vi "Main.vi"(11 "Module Admin":refnum<class "Delacor_lib_QMH_Module Admin.lvclass">) -> ()   [LabVIEW 2020, in "ATM.lvlib"]
doc: "This template is based off of the Queued Message Handler design pattern and the Queued Message Handler project template that ships with LabVIEW.\n\nThe main difference is that the queue is private to this module and communication between modules is performed via Broadcast and Request events.\n\nRequest events are wrapped in public API methods and are handled in the Event Handling Loop (EHL) of this VI. Any module can register for Broadcast events sent by this module. The EHL generates messages based on user interface actions.\n\nThe Message Handling Loop (MHL) processes messages generated by the EHL, or by other messages. The messages are string values, so new messages can be added easily to the Message Cases case structure in the MHL. Each message cluster can also provide an optional value for Message Data, which is a variant that can be converted to whatever message-specific data is required.\n_____\nBased on DQMH Dev Tools: Project Template 7.1.0.1503."
uses:
  ATM.lvlib
  <vilib>/Delacor/Delacor QMH/Libraries/Message Queue_class/Delacor_lib_QMH_Message Queue.lvclass
  Module Data--cluster.ctl
  <vilib>/Utility/miscctls.llb/LVPointTypeDef.ctl
  <vilib>/Delacor/Delacor QMH/Libraries/Message Queue_class/Delacor_lib_QMH_Enqueue Message (Single).vi
  Stop Argument--cluster.ctl
  <vilib>/Delacor/Delacor QMH/Libraries/Module Admin_class/Delacor_lib_QMH_Module Admin.lvclass
  Update ATM Messages Argument--cluster.ctl
  Account Info -- cluster.ctl
  Deposit Introduced Argument--cluster.ctl
  Accounts Info -- cluster.ctl
  Check Withdrawal Argument--cluster.ctl
  <vilib>/ErrorRing/Error Ring.xnode
panel:
  in  "Enter":bool
  in  "User Input":string
  in  "Right Buttons":T1
  out "Right Menu":T2
  in  "Left Buttons":T1
  out "Left Menu":T2
  in  "Card Simulator":bool
  out "ATM Messages":string
  out "error out":errorcluster
  out "Status":string
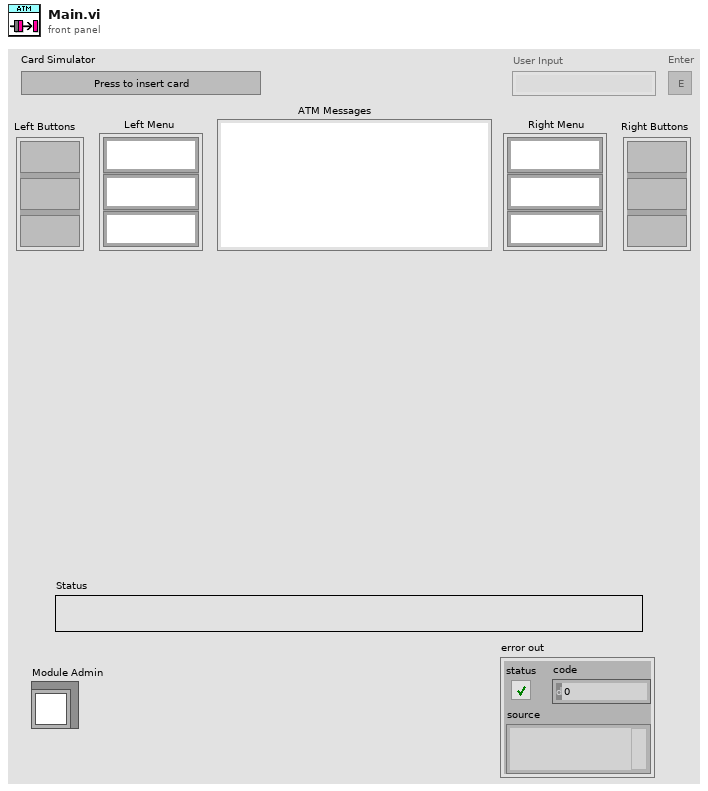
[diagram p1: front panel]
types:
  T1 = cluster{"Func Button":bool, "Func Button 2":bool, "Func Button 3":bool}
  T2 = cluster{"RFS String":string, "RFS String 2":string, "RFS String 3":string}
  T3 = typedef "ATM.lvlib/Request Events--cluster.ctl" = cluster{"Stop Module":refnum<user-event>, "Show Panel":refnum<user-event>, "Hide Panel":refnum<user-event>, "Get Module Execution Status":refnum<user-event>, "Show Diagram":refnum<user-event>, "Private.Set Up Controls":refnum<user-event>, "Private.Update ATM Messages":refnum<user-event>, "Private.Start Timeout":refnum<user-event>, "Private.Set Up Accounts File":refnum<user-event>, "Private.Verification OK":refnum<user-event>, "Private.Session Timed Out":refnum<user-event>, "Private.Verification NOK":refnum<user-event>, "Private.Stop Timeout":refnum<user-event>, "Private.Deposit Introduced":refnum<user-event>, "Private.Save Account":refnum<user-event>, "Private.Check Withdrawal":refnum<user-event>, "Testing - Update ATM Messages":refnum<user-event>, "Testing - Generate File Not Found Error":refnum<user-event>, "Testing - Enable All Elements in FP":refnum<user-event>, "Testing - Disable All Elements in FP":refnum<user-event>}
  T4 = typedef "ATM.lvlib/Module Data--cluster.ctl" = cluster{"Status":string, "User Input":string, "Verification OK?":bool, "User Input ref":refnum<vi>, "Left Buttons ref":refnum<vi>, "Right Buttons ref":refnum<vi>, "Enter ref":refnum<vi>, "Right Menu ref":refnum<vi>, "Left Menu ref":refnum<vi>, "Card Simulator":refnum<vi>, "Accounts.txt file name":string, "Accounts.txt file path":path, "Account Info":T5, "Accounts info":T6, "Pressed Button":string, "Index of Account":i32}
  T5 = typedef "ATM.lvlib/Account Info -- cluster.ctl" = cluster{"Account Number":string, "Name":string, "Surname":string, "Remaining Money":i32}
  T6 = typedef "ATM.lvlib/Accounts Info -- cluster.ctl" = T5[]
  T7 = typedef "ATM.lvlib/Check Withdrawal Argument--cluster.ctl" = cluster{"Withdraw Money":i32}
  T8 = typedef "ATM.lvlib/Deposit Introduced Argument--cluster.ctl" = cluster{"Deposit Money":u32}
  T9 = typedef "ATM.lvlib/Update ATM Messages Argument--cluster.ctl" = cluster{"ATM Messages":string}
  T10 = enum32{"invalid lock state", "Not Locked", "Locked (No Password)", "Password-protected"}
  T11 = typedef "ATM.lvlib/Stop Argument--cluster.ctl" = cluster{"Origin":string, "Exit via Stop Module Req?":bool, "Wait for Module to stop?":bool}
  T12 = typedef "LVPointTypeDef.ctl" = cluster{"Horizontal":i16, "Vertical":i16}
  T13 = enum32{"Invalid", "Standard", "Closed", "Hidden", "Minimized", "Maximized"}
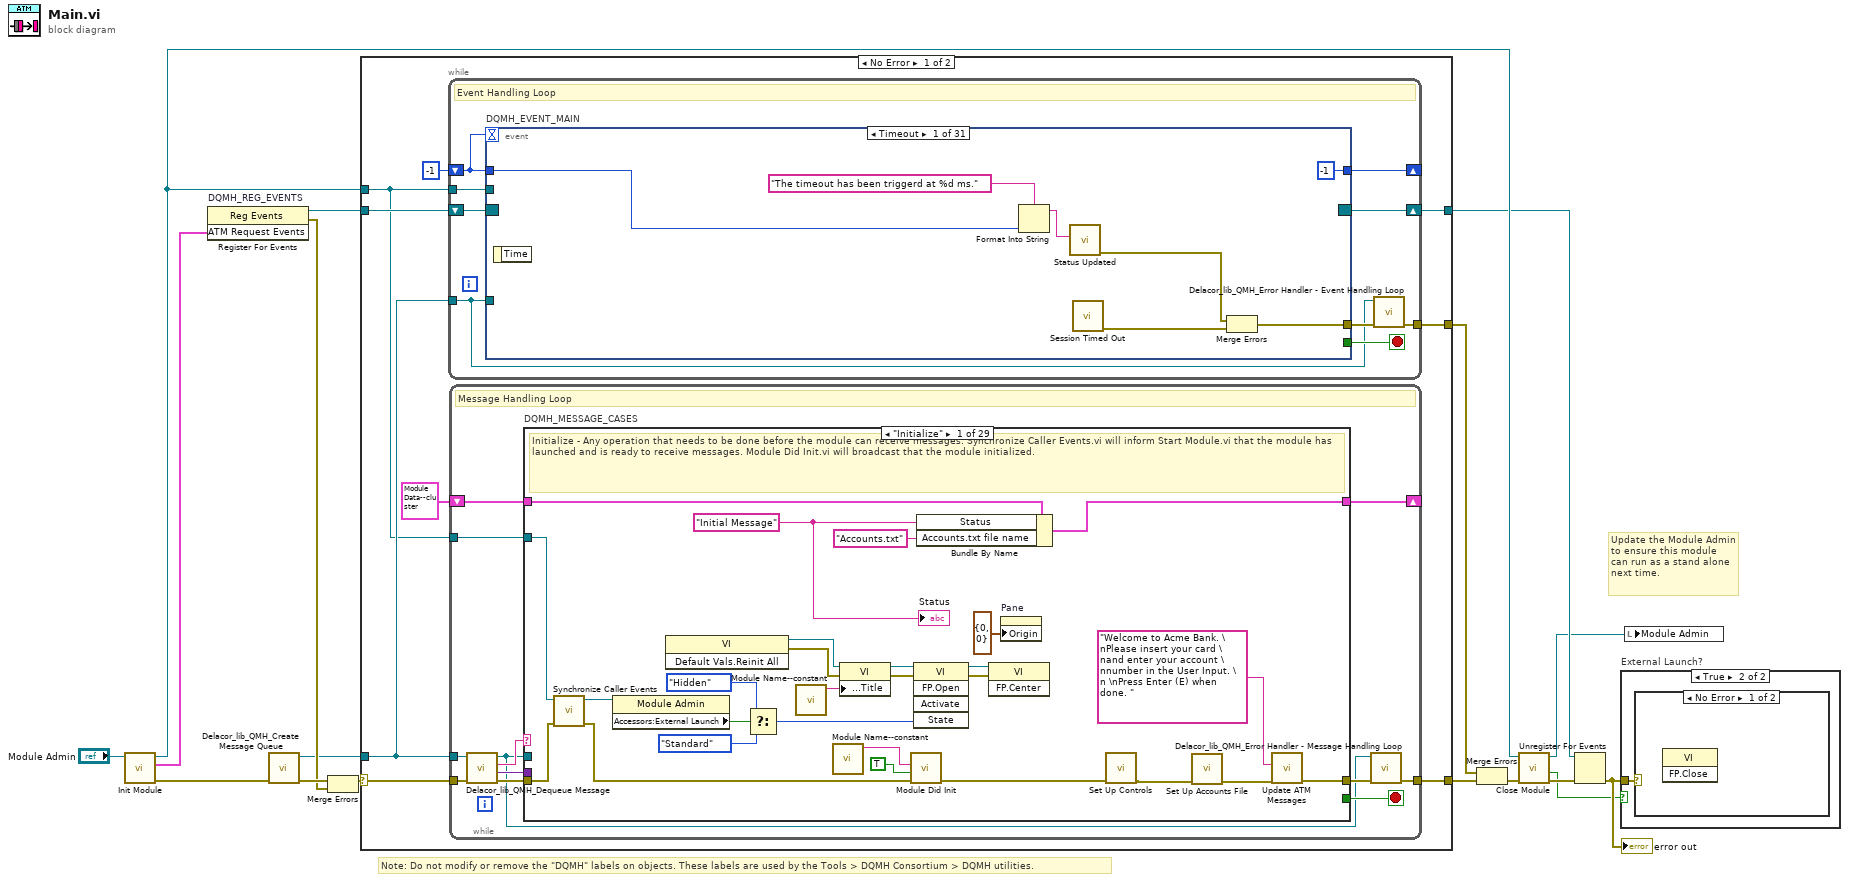
[diagram p0: block diagram]
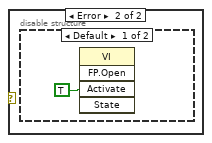
[diagram p3: hidden frame]
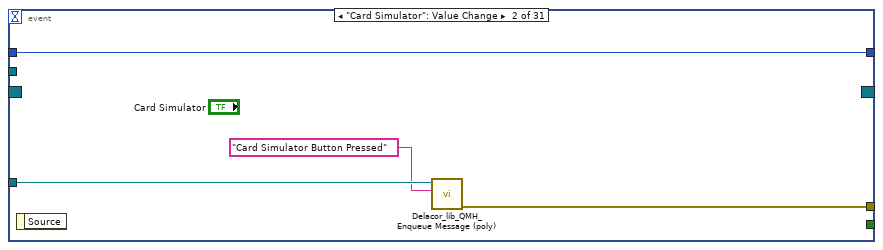
[diagram p5: hidden frame]
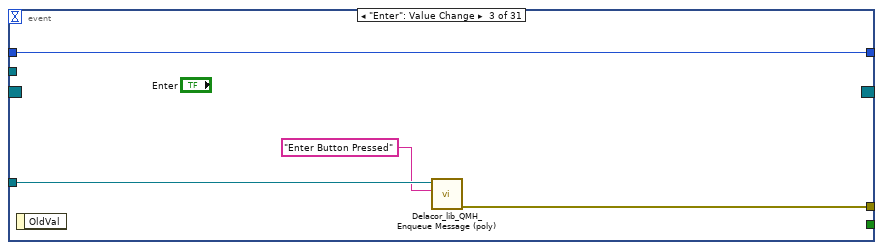
[diagram p6: hidden frame]
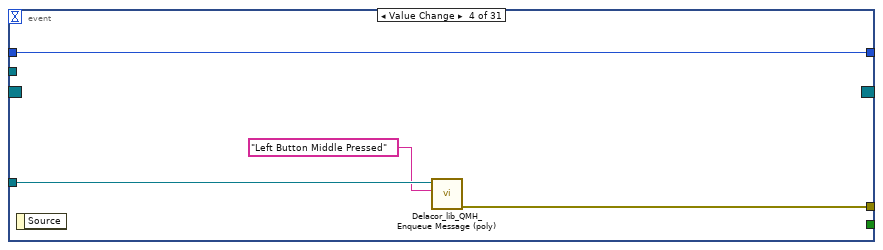
[diagram p7: hidden frame]
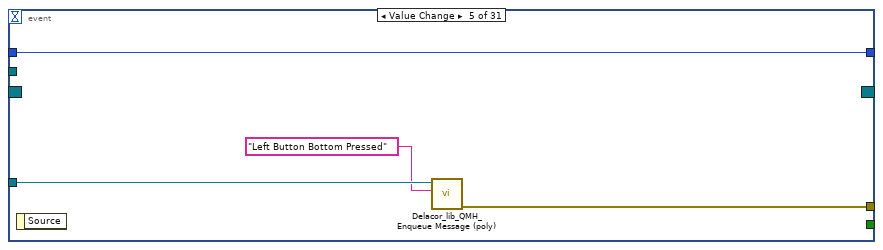
[diagram p8: hidden frame]
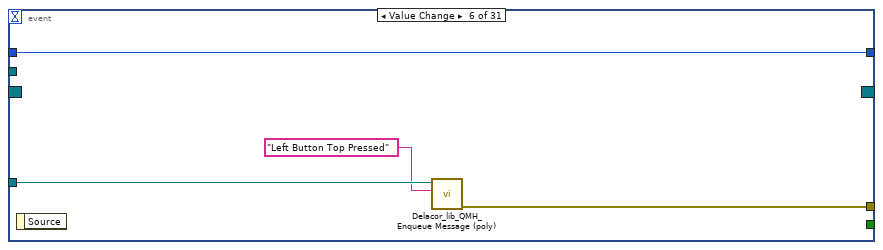
[diagram p9: hidden frame]
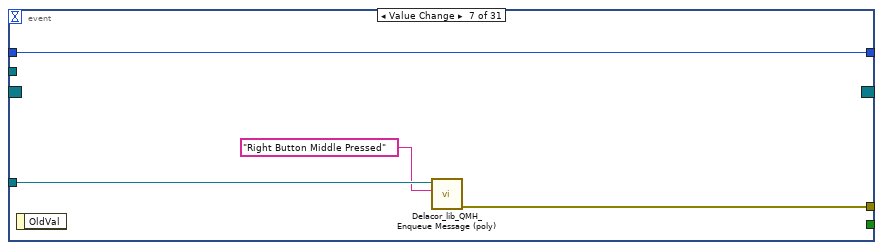
[diagram p10: hidden frame]
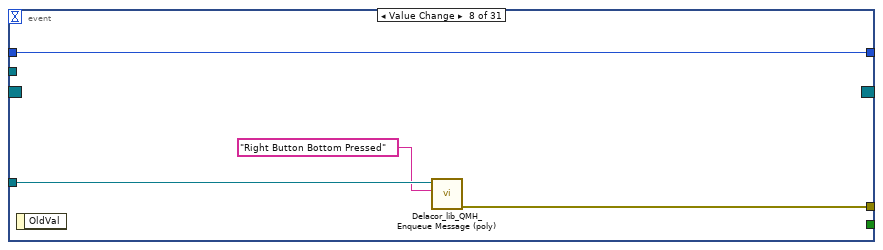
[diagram p11: hidden frame]
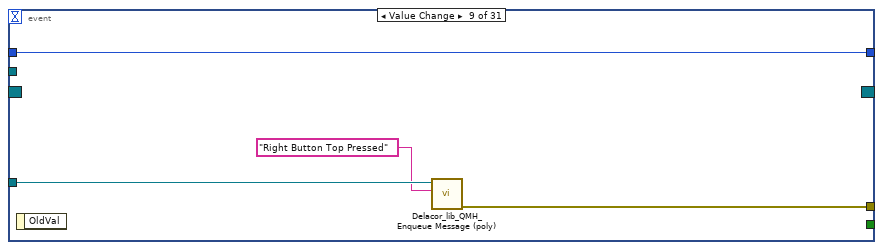
[diagram p12: hidden frame]
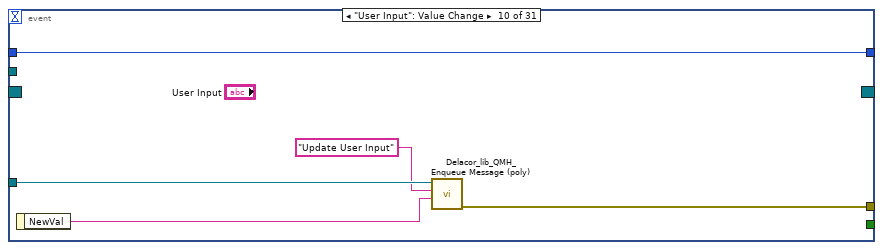
[diagram p13: hidden frame]
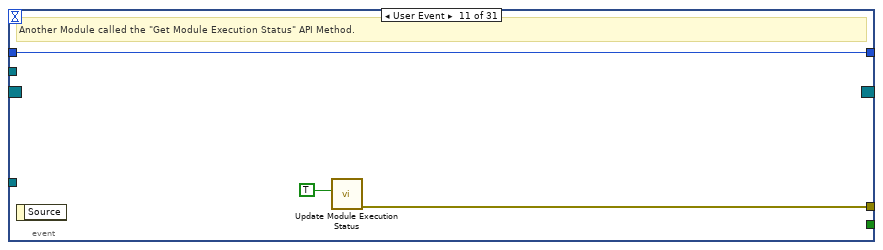
[diagram p14: hidden frame]
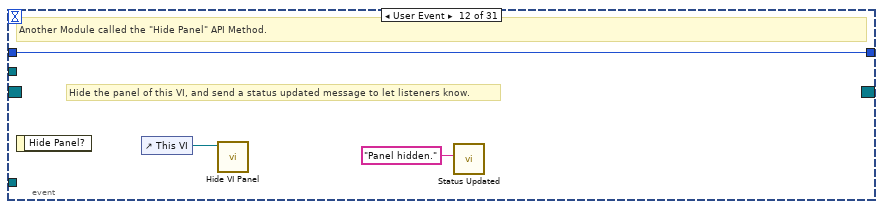
[diagram p15: hidden frame]
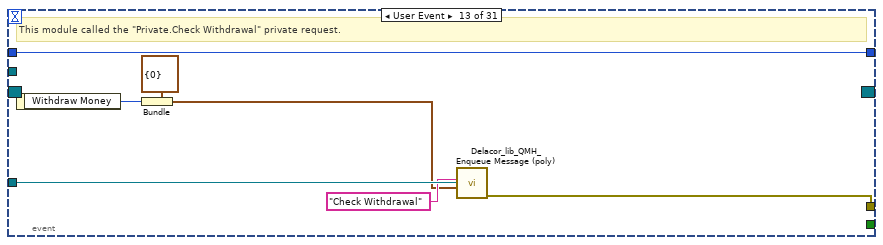
[diagram p16: hidden frame]
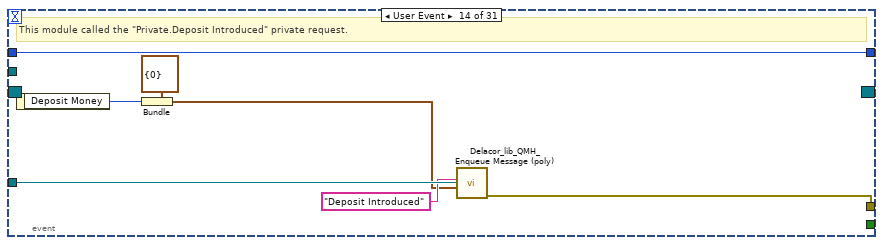
[diagram p17: hidden frame]
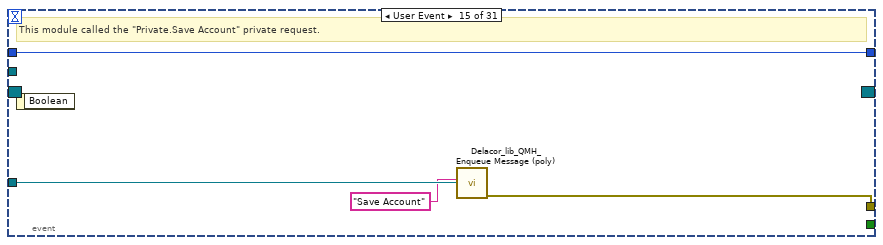
[diagram p18: hidden frame]
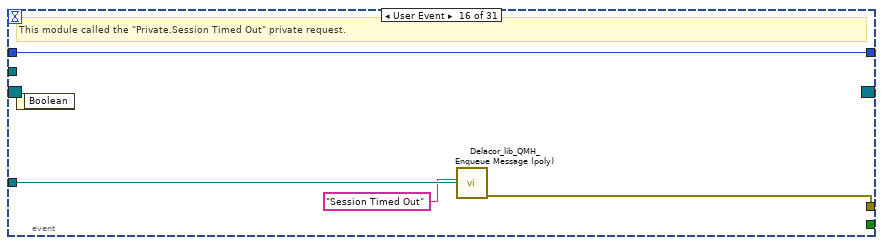
[diagram p19: hidden frame]
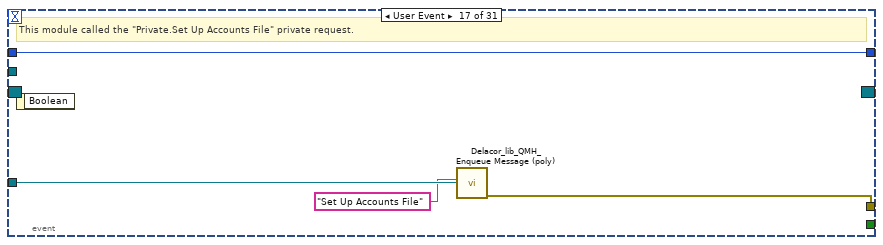
[diagram p20: hidden frame]
diagram:
  # "Note: Do not modify or remove the \"DQMH\" labels on objects. These labels are used by the Tools > DQMH Consortium > DQMH utilities."
  # "Update the Module Admin to ensure this module can run as a stand alone next time."
  n1 = call "Init Module.vi"("Singleton Module Admin in"="Module Admin") -> ("error out"=w16:errorcluster, "ATM Request Events"=w5:T3, "Singleton Module Admin out"=w8:refnum<class "Delacor_lib_QMH_Module Admin.lvclass">)  [unwired: 8 in]
  n2 = register-events "DQMH_REG_EVENTS"(w5) -> (reference out=w6:refnum<event-registration>, error out=w9:errorcluster)  [unwired: 2 in]
  n3 = call <vilib>:"Delacor_lib_QMH_Create Message Queue.vi"("error in"=w16) -> ("error out"=w11:errorcluster, "Message Queue"=w4:refnum<class "Delacor_lib_QMH_Message Queue.lvclass">)  [unwired: 9 in]
  n4 = Merge Errors(w11, w9) -> (w10:errorcluster)
  n5 = case shown="No Error" w10 {
    selector: w10 -> [w24 w589]
    tunnel: [w26 w588] -> w17
    tunnel: [w23 w587] -> w7
    tunnel: w6 -> [w21 w587]
    tunnel: w4 -> [w20 w582]
    tunnel: [w25 _] -> w14
    tunnel: w8 -> [w19 w583]
    frame No Error {
      n6 = while {
        tunnel: w20 -> [w29]
        shift-right: [w32] -> w23
        shift-left: w21 -> [w33]
        tunnel: [w34] -> w25
        tunnel: w19 -> [w30]
        shift-right: [w28] -> _
        shift-left: -1 ("Timeout Time") -> [w27]
        stop <- w31 stop-if-true
        # "Event Handling Loop"
        n7 = event "DQMH_EVENT_MAIN" shown="[0] Timeout" {
          selector: w33 -> [_ _ _ _ _ _ _ _ _ _ _ _ _ _ _ _ _ _ _ _ _ _ _ _ _ _ _ _ _ _ _]
          dyn-events: [_ _ _ _ _ _ _ _ _ _ _ _ _ _ _ _ _ _ _ _ _ _ _ _ _ _ _ _ _ _ _] -> w32
          timeout: w27 -> [_ _ _ _ _ _ _ _ _ _ _ _ _ _ _ _ _ _ _ _ _ _ _ _ _ _ _ _ _ _ _]
          tunnel: [_ _ _ _ _ _ _ _ _ _ _ _ _ _ _ _ _ _ _ _ _ _ _ _ _ TRUE ("Discard?") _ _ _ _ _] -> w31
          tunnel: w29 -> [_ w46 w50 w54 w58 w62 w66 w70 w74 w79 _ _ w91 w98 w102 w106 w111 w115 _ _ w128 w131 w136 _ _ w158 w165 w169 w173 w177 w182]
          tunnel: [w37 w44 w48 w52 w56 w60 w64 w68 w72 w77 w82 _ w86 w93 w100 w104 w109 w113 w120 _ w123 w129 w134 _ _ w161 w163 w167 w171 w175 w184] -> w35
          tunnel: w30 -> [_ _ _ _ _ _ _ _ _ _ _ _ _ _ _ _ _ _ _ _ _ _ _ _ _ _ _ _ _ _ w181]
          tunnel: [-1 ("Timeout Time") w43 w47 w51 w55 w59 w63 w67 w71 w75 w80 w83 w92 w99 w103 w107 w108 w112 w118 -1 ("Timeout Time") w122 w132 w133 w137 w147 w150 w166 w170 w174 w178 w179] -> w28
          tunnel: w27 -> [w39 w43 w47 w51 w55 w59 w63 w67 w71 w75 w80 w83 w92 w99 w103 w107 w108 w112 _ _ w122 w132 w133 w137 w147 w150 w166 w170 w174 w178 w179]
          event Timeout {
            n8 = event-data() -> ()  [unwired: 1 in, 1 out]
            n9 = Format Into String(format string="The timeout has been triggerd at %d ms.", w39) -> (resulting string=w38:string)  [unwired: 2 in, 1 out]
            n10 = call "Status Updated.vi"("Status"=w38) -> ("error out"=w36:errorcluster)  [unwired: 10 in]
            n11 = call "Session Timed Out.vi"() -> ("error out"=w41:errorcluster)  [unwired: 11 in]
            n12 = Merge Errors(w36, w41) -> (w37:errorcluster)
          }
          event "Card Simulator": Value Change {
            n13 = event-data() -> ()  [unwired: 1 in, 1 out]
            n14 = call-poly <vilib>:"Delacor_lib_QMH_Enqueue Message (poly).vi"("Message"="Card Simulator Button Pressed", "Message Queue in"=w46) -> ("error out"=w44:errorcluster)  [unwired: 8 in, 1 out]
          }
          event "Enter": Value Change {
            n15 = event-data() -> ()  [unwired: 1 in, 1 out]
            n16 = call-poly <vilib>:"Delacor_lib_QMH_Enqueue Message (poly).vi"("Message"="Enter Button Pressed", "Message Queue in"=w50) -> ("error out"=w48:errorcluster)  [unwired: 8 in, 1 out]
          }
          event "Left Buttons.Func Button 2": Value Change {
            n17 = event-data() -> ()  [unwired: 1 in, 1 out]
            n18 = call-poly <vilib>:"Delacor_lib_QMH_Enqueue Message (poly).vi"("Message"="Left Button Middle Pressed", "Message Queue in"=w54) -> ("error out"=w52:errorcluster)  [unwired: 8 in, 1 out]
          }
          event "Left Buttons.Func Button 3": Value Change {
            n19 = event-data() -> ()  [unwired: 1 in, 1 out]
            n20 = call-poly <vilib>:"Delacor_lib_QMH_Enqueue Message (poly).vi"("Message"="Left Button Bottom Pressed", "Message Queue in"=w58) -> ("error out"=w56:errorcluster)  [unwired: 8 in, 1 out]
          }
          event "Left Buttons.Func Button": Value Change {
            n21 = event-data() -> ()  [unwired: 1 in, 1 out]
            n22 = call-poly <vilib>:"Delacor_lib_QMH_Enqueue Message (poly).vi"("Message"="Left Button Top Pressed", "Message Queue in"=w62) -> ("error out"=w60:errorcluster)  [unwired: 8 in, 1 out]
          }
          event "Right Buttons.Func Button 2": Value Change {
            n23 = event-data() -> ()  [unwired: 1 in, 1 out]
            n24 = call-poly <vilib>:"Delacor_lib_QMH_Enqueue Message (poly).vi"("Message"="Right Button Middle Pressed", "Message Queue in"=w66) -> ("error out"=w64:errorcluster)  [unwired: 8 in, 1 out]
          }
          event "Right Buttons.Func Button 3": Value Change {
            n25 = event-data() -> ()  [unwired: 1 in, 1 out]
            n26 = call-poly <vilib>:"Delacor_lib_QMH_Enqueue Message (poly).vi"("Message"="Right Button Bottom Pressed", "Message Queue in"=w70) -> ("error out"=w68:errorcluster)  [unwired: 8 in, 1 out]
          }
          event "Right Buttons.Func Button": Value Change {
            n27 = event-data() -> ()  [unwired: 1 in, 1 out]
            n28 = call-poly <vilib>:"Delacor_lib_QMH_Enqueue Message (poly).vi"("Message"="Right Button Top Pressed", "Message Queue in"=w74) -> ("error out"=w72:errorcluster)  [unwired: 8 in, 1 out]
          }
          event "User Input": Value Change {
            n29 = event-data() -> ("NewVal"=w76:string)  [unwired: 1 in]
            n30 = call-poly <vilib>:"Delacor_lib_QMH_Enqueue Message (poly).vi"("Message Data"=w76, "Message"="Update User Input", "Message Queue in"=w79) -> ("error out"=w77:errorcluster)  [unwired: 7 in, 1 out]
          }
          event User Event {
            # "Another Module called the \"Get Module Execution Status\" API Method."
            n31 = event-data() -> ()  [unwired: 1 in, 1 out]
            n32 = call "Update Module Execution Status.vi"("Running?"=TRUE) -> ("error out"=w82:errorcluster)  [unwired: 10 in]
          }
          event User Event {
            # "Hide the panel of this VI, and send a status updated message to let listeners know."
            # "Another Module called the \"Hide Panel\" API Method."
            n33 = event-data() -> ()  [unwired: 1 in, 1 out]
            n34 = control-ref of="This VI"() -> (w85:refnum<vi>)
            n35 = call "Hide VI Panel.vi"("VI"=w85) -> ()  [unwired: 10 in, 1 out]
            n36 = call "Status Updated.vi"("Status"="Panel hidden." ("format string")) -> ()  [unwired: 10 in, 1 out]
          }
          event User Event {
            # "This module called the \"Private.Check Withdrawal\" private request."
            n37 = event-data() -> ("Withdraw Money"=w87:i32)  [unwired: 1 in]
            n38 = Bundle(cluster=T7 {"Withdraw Money"=0} ("Check Withdrawal Argument"), "Withdraw Money"=w87) -> (w88:T7)
            n39 = call-poly <vilib>:"Delacor_lib_QMH_Enqueue Message (poly).vi"("Message Data"=w88, "Message"="Check Withdrawal", "Message Queue in"=w91) -> ("error out"=w86:errorcluster)  [unwired: 7 in, 1 out]
          }
          event User Event {
            # "This module called the \"Private.Deposit Introduced\" private request."
            n40 = event-data() -> ("Deposit Money"=w94:u32)  [unwired: 1 in]
            n41 = Bundle(cluster=T8 {"Deposit Money"=0} ("Deposit Introduced Argument"), "Deposit Money"=w94) -> (w95:T8)
            n42 = call-poly <vilib>:"Delacor_lib_QMH_Enqueue Message (poly).vi"("Message Data"=w95, "Message"="Deposit Introduced", "Message Queue in"=w98) -> ("error out"=w93:errorcluster)  [unwired: 7 in, 1 out]
          }
          event User Event {
            # "This module called the \"Private.Save Account\" private request."
            n43 = event-data() -> ()  [unwired: 1 in, 1 out]
            n44 = call-poly <vilib>:"Delacor_lib_QMH_Enqueue Message (poly).vi"("Message"="Save Account", "Message Queue in"=w102) -> ("error out"=w100:errorcluster)  [unwired: 8 in, 1 out]
          }
          event User Event {
            # "This module called the \"Private.Session Timed Out\" private request."
            n45 = event-data() -> ()  [unwired: 1 in, 1 out]
            n46 = call-poly <vilib>:"Delacor_lib_QMH_Enqueue Message (poly).vi"("Message"="Session Timed Out", "Message Queue in"=w106) -> ("error out"=w104:errorcluster)  [unwired: 8 in, 1 out]
          }
          event User Event {
            # "This module called the \"Private.Set Up Accounts File\" private request."
            n47 = event-data() -> ()  [unwired: 1 in, 1 out]
            n48 = call-poly <vilib>:"Delacor_lib_QMH_Enqueue Message (poly).vi"("Message"="Set Up Accounts File", "Message Queue in"=w111) -> ("error out"=w109:errorcluster)  [unwired: 8 in, 1 out]
          }
          event User Event {
            # "This module called the \"Private.Set Up Controls\" private request."
            n49 = event-data() -> ()  [unwired: 1 in, 1 out]
            n50 = call-poly <vilib>:"Delacor_lib_QMH_Enqueue Message (poly).vi"("Message"="Set Up Controls", "Message Queue in"=w115) -> ("error out"=w113:errorcluster)  [unwired: 8 in, 1 out]
          }
          event User Event {
            # "This module called the \"Private.Start Timeout\" private request."
            n51 = event-data() -> ("Timeout Time"=w118:i32)  [unwired: 1 in]
            n52 = Format Into String(format string="A Timeout has been launched with a value of %d ms.", w118) -> (resulting string=w117:string, error out=w116:errorcluster)  [unwired: 2 in]
            n53 = call "Status Updated.vi"("error in"=w116, "Status"=w117) -> ("error out"=w120:errorcluster)  [unwired: 9 in]
          }
          event User Event {
            # "This module called the \"Private.Stop Timeout\" private request."
            n54 = event-data() -> ()  [unwired: 1 in, 1 out]
          }
          event User Event {
            # "This module called the \"Private.Update ATM Messages\" private request."
            n55 = event-data() -> ("ATM Messages"=w124:string)  [unwired: 1 in]
            n56 = Bundle(cluster=T9 {"ATM Messages"=""} ("Update ATM Messages Argument"), "ATM Messages"=w124) -> (w125:T9)
            n57 = call-poly <vilib>:"Delacor_lib_QMH_Enqueue Message (poly).vi"("Message Data"=w125, "Message"="Update ATM Messages", "Message Queue in"=w128) -> ("error out"=w123:errorcluster)  [unwired: 7 in, 1 out]
          }
          event User Event {
            # "This module called the \"Private.Verification NOK\" private request."
            n58 = event-data() -> ()  [unwired: 1 in, 1 out]
            n59 = call-poly <vilib>:"Delacor_lib_QMH_Enqueue Message (poly).vi"("Message"="Verification NOK", "Message Queue in"=w131) -> ("error out"=w129:errorcluster)  [unwired: 8 in, 1 out]
          }
          event User Event {
            # "This module called the \"Private.Verification OK\" private request."
            n60 = event-data() -> ()  [unwired: 1 in, 1 out]
            n61 = call-poly <vilib>:"Delacor_lib_QMH_Enqueue Message (poly).vi"("Message"="Verification OK", "Message Queue in"=w136) -> ("error out"=w134:errorcluster)  [unwired: 8 in, 1 out]
          }
          event User Event {
            # "Another Module called the \"Show Diagram\" API Method. This event is used for debugging."
            n62 = event-data() -> ()  [unwired: 1 in, 1 out]
            n63 = disable-structure shown="RUN_TIME_ENGINE==False" {
              frame condition #0 (active) {
                # "functionality not available in exe"
                n64 = invoke on="Invoke Node" class="VI" method="Lock State.Get"() -> (error out=w143:errorcluster, "Get Lock State"=w142:T10, "pwd in cache"=w139:bool)  [unwired: 4 in, 1 out]
                n65 = Equal?(x=T10."Password-protected", y=w142) -> (x = y?=w140:bool)
                n66 = Compound Arithmetic op=AND(w140, invert w139) -> (w138:bool)
                n67 = case shown="False" w138 {
                  tunnel: w143 -> [w146 _]
                  frame False {
                    n68 = property on="Property Node" class="VI"(error in=w146, "BDWin.Open"=TRUE ("Block Diagram Window:Open")) -> ()  [unwired: 1 in, 2 out]
                    n69 = call "Status Updated.vi"("Status"="Block Diagram shown." ("format string")) -> ()  [unwired: 10 in, 1 out]
                  }
                  frame True {
                    # "Password-protected VI, and the password is not in the cache. Do not show the diagram."
                  }
                }
              }
              frame condition #1 {
              }
            }
          }
          event User Event {
            # "Show the panel of this VI, and send a status updated message to let listeners know."
            # "Another Module called the \"Show Panel\" API Method."
            n70 = event-data() -> ()  [unwired: 1 in, 1 out]
            n71 = control-ref of="This VI"() -> (w149:refnum<vi>)
            n72 = call "Open VI Panel.vi"("VI"=w149) -> ()  [unwired: 10 in, 1 out]
            n73 = call "Status Updated.vi"("Status"="Panel shown." ("format string")) -> ()  [unwired: 10 in, 1 out]
          }
          event User Event {
            # "The Stop Module Event can get fired from the Exit message in the MHL. The queue gets destroyed in that case. If the queue no longer exists, the Enqueue Exit as a priority message will return error 1. It is safe to ignore, because the module is already exiting."
            # "Another Module called the \"Stop Module\" API Method  or the Message Handling Loop below."
            n74 = event-data() -> ("Origin"=w157:string, "Exit via Stop Module Req?"=w153:bool, "Wait for Module to stop?"=w152:bool)  [unwired: 1 in]
            n75 = local write "Status"(w157) -> ()
            n76 = Bundle By Name(cluster=T11 {"Origin"="", "Exit via Stop Module Req?"=FALSE, "Wait for Module to stop?"=FALSE} ("Stop Argument"), "Exit via Stop Module Req?"=w153, "Wait for Module to stop?"=w152) -> (w151:T11)
            n77 = call-poly <vilib>:"Delacor_lib_QMH_Enqueue Message (poly).vi"("Priority Message? (F)"=TRUE, "Message Data"=w151, "Message"="Exit", "Message Queue in"=w158) -> ("error out"=w162:errorcluster)  [unwired: 6 in, 1 out]
            n78 = call <vilib>:"Clear Errors.vi"("error in (no error)"=w162, "specific error code to clear (0: all)"=1) -> ("error out"=w161:errorcluster)  [unwired: 4 in, 1 out]
          }
          event User Event {
            # "Another Module called the \"Testing - Disable All Elements in FP\" API Method."
            n79 = event-data() -> ()  [unwired: 1 in, 1 out]
            n80 = call-poly <vilib>:"Delacor_lib_QMH_Enqueue Message (poly).vi"("Message"="Testing - Disable All Elements in FP", "Message Queue in"=w165) -> ("error out"=w163:errorcluster)  [unwired: 8 in, 1 out]
          }
          event User Event {
            # "Another Module called the \"Testing - Enable All Elements in FP\" API Method."
            n81 = event-data() -> ()  [unwired: 1 in, 1 out]
            n82 = call-poly <vilib>:"Delacor_lib_QMH_Enqueue Message (poly).vi"("Message"="Testing - Enable All Elements in FP", "Message Queue in"=w169) -> ("error out"=w167:errorcluster)  [unwired: 8 in, 1 out]
          }
          event User Event {
            # "Another Module called the \"Testing - Generate File Not Found Error\" API Method."
            n83 = event-data() -> ()  [unwired: 1 in, 1 out]
            n84 = call-poly <vilib>:"Delacor_lib_QMH_Enqueue Message (poly).vi"("Message"="Testing - Generate File Not Found Error", "Message Queue in"=w173) -> ("error out"=w171:errorcluster)  [unwired: 8 in, 1 out]
          }
          event User Event {
            # "Another Module called the \"Testing - Update ATM Messages\" API Method."
            n85 = event-data() -> ()  [unwired: 1 in, 1 out]
            n86 = call-poly <vilib>:"Delacor_lib_QMH_Enqueue Message (poly).vi"("Message"="Testing - Update ATM Messages", "Message Queue in"=w177) -> ("error out"=w175:errorcluster)  [unwired: 8 in, 1 out]
          }
          event Panel Close? {
            w183 = TRUE  # Discard the event, the MHL is responsible for closing and stopping this VI.
            # "Hide the panel or send the 'Exit' message if the user clicks the 'X' on the module main VI panel."
            n87 = event-data() -> ()  [unwired: 1 in, 1 out]
            n88 = property on="Property Node" class="Module Admin"(reference=w181) -> ("Accessors:External Launch"=w180:bool)  [unwired: 1 in, 2 out]
            n89 = case shown="True" w180 {
              tunnel: w182 -> [_ w190]
              tunnel: [_ w191] -> w184
              frame True {
                # "If externally launched, clicking the 'X' hides the panel, but doesn't close it."
                n90 = control-ref of="This VI"() -> (w187:refnum<vi>)
                n91 = call "Hide VI Panel.vi"("VI"=w187) -> ("error out"=w185:errorcluster)  [unwired: 10 in]
                n92 = call "Status Updated.vi"("error in"=w185, "Status"="Panel hidden." ("format string")) -> ()  [unwired: 9 in, 1 out]
              }
              frame False {
                # "If run as a stand-alone VI, clicking the panel 'X' stops the VI."
                n93 = call-poly <vilib>:"Delacor_lib_QMH_Enqueue Message (poly).vi"("Priority Message? (F)"=TRUE, "Message"="Exit", "Message Queue in"=w190) -> ("error out"=w191:errorcluster)  [unwired: 7 in, 1 out]
              }
            }
            n94 = event-data ("Event Filter Node")("Discard?"=w183) -> ()  [unwired: 1 in, 1 out]
          }
        }
        n95 = call-dynamic "Delacor_lib_QMH_Error Handler - Event Handling Loop.vi"("error in"=w35, "Message Queue in"=w29) -> ("dup error in"=w34:errorcluster)  [unwired: 8 in, 1 out]
      }
      n96 = while {
        tunnel: w20 -> [w192]
        shift-right: [w200] -> _
        shift-left: T4 {"Status"="", "User Input"="", "Verification OK?"=FALSE, "User Input ref"=refnum, "Left Buttons ref"=refnum, "Right Buttons ref"=refnum, "Enter ref"=refnum, "Right Menu ref"=refnum, "Left Menu ref"=refnum, "Card Simulator"=refnum, "Accounts.txt file name"="", "Accounts.txt file path"=path "", "Account Info"={"Account Number"="", "Name"="", "Surname"="", "Remaining Money"=0}, "Accounts info"=[], "Pressed Button"="", "Index of Account"=0} ("Data Cluster") -> [w201]
        tunnel: w24 -> [w203]
        tunnel: [w195] -> w26
        tunnel: w19 -> [w196]
        stop <- w199 stop-if-true
        # "Message Handling Loop"
        n97 = call-dynamic "Delacor_lib_QMH_Dequeue Message.vi"("error in"=w203, "Message Queue in"=w192) -> ("error out"=w202:errorcluster, "Message Data"=w197:variant, "Message"=w198:string, "Message Queue out"=w193:refnum<class "Delacor_lib_QMH_Message Queue.lvclass">)  [unwired: 6 in]
        n98 = case "DQMH_MESSAGE_CASES" shown="\"Initialize\"" w198 {
          selector: w198 -> [_ _ _ _ _ _ _ _ _ _ _ _ w367 w389 w399 w412 w421 _ _ _ _ _ _ _ _ _ _ _ w577]
          tunnel: w193 -> [_ _ _ _ _ _ _ _ _ _ _ _ _ _ _ _ _ _ _ _ _ _ _ _ _ _ w542 w565 _]
          tunnel: w202 -> [w228 w232 w247 w253 w264 w277 w292 w298 w301 w308 w322 w365 w378 w387 w398 w410 w418 w444 w453 w468 w490 w495 w499 w515 w531 w538 w549 w571 w580]
          tunnel: [w210 w232 w238 w252 w262 w279 w295 w297 w301 w306 w312 w358 w370 w391 w401 w414 w419 w428 w448 w462 w489 w492 w498 w514 w530 w538 w545 w566 w581] -> w194
          tunnel: w201 -> [w218 w231 w249 w257 w263 w289 w294 w299 w300 w307 w321 w364 w376 w384 w396 w407 w420 w440 w452 w459 w488 w496 w500 w513 w529 w537 w544 w564 w578]
          tunnel: [w217 w231 w248 w256 w263 w273 w294 w299 w300 w304 w318 w364 w368 w390 w400 w413 w422 w438 w447 w457 w488 w496 w500 w513 w529 w537 w544 w564 w578] -> w200
          tunnel: [_ _ _ _ _ _ _ _ _ _ _ _ _ _ _ _ _ _ _ _ _ _ _ _ _ _ _ w563 _] -> w199
          tunnel: w197 -> [_ _ _ _ w261 _ _ _ _ w305 _ _ _ _ _ _ _ w443 _ w467 _ _ _ _ _ _ w543 w562 _]
          tunnel: w196 -> [w219 _ _ _ _ _ _ _ _ _ _ _ _ _ _ _ _ _ _ _ _ _ _ _ _ _ w541 w557 _]
          frame "Initialize" {
            w213 = "Initial Message" ("Initial Message")
            # "Initialize - Any operation that needs to be done before the module can receive messages. Synchronize Caller Events.vi will inform Start Module.vi that the module has launched and is ready to receive messages. Module Did Init.vi will broadcast that the module initialized."
            n99 = call "Synchronize Caller Events.vi"("error in"=w228, "Singleton Module Admin in"=w219) -> ("error out"=w227:errorcluster, "Singleton Module Admin out"=w214:refnum<class "Delacor_lib_QMH_Module Admin.lvclass">)  [unwired: 8 in]
            n100 = property on="Property Node" class="Module Admin"(reference=w214) -> ("Accessors:External Launch"=w223:bool)  [unwired: 1 in, 2 out]
            n101 = invoke class="VI" method="Default Vals.Reinit All"() -> (reference out=w208:refnum<vi>, error out=w207:errorcluster)  [unwired: 3 in, 1 out]
            n102 = Select(t=T13."Hidden" ("State"), s=w223, f=T13."Standard" ("State")) -> (s? t:f=w220:T13)
            n103 = call "Module Name--constant.vi"() -> ("Module Name"=w226:string)  [unwired: 11 in]
            n104 = call "Module Name--constant.vi"() -> ("Module Name"=w215:string)  [unwired: 11 in]
            n105 = property on="Property Node" class="VI"(reference=w208, error in=w207, "Front Panel.Title"=w226) -> (reference out=w225:refnum<vi>, error out=w230:errorcluster)
            n106 = call "Module Did Init.vi"("error in"=w227, "Initialized?"=TRUE, "Origin"=w215) -> ("error out"=w211:errorcluster)  [unwired: 8 in]
            n107 = invoke on="Invoke Node" class="VI" method="FP.Open"(reference=w225, error in=w230, "State"=w220) -> (reference out=w224:refnum<vi>, error out=w229:errorcluster)  [unwired: 2 in, 3 out]
            n108 = Bundle By Name(cluster=w218, "Status"=w213, "Accounts.txt file name"="Accounts.txt") -> (w217:T4)
            n109 = invoke on="Invoke Node" class="VI" method="FP.Center"(reference=w224, error in=w229) -> ()  [unwired: 1 in, 3 out]
            n110 = property on="Pane" class="Pane"("Origin"=T12 {"Horizontal"=0, "Vertical"=0}) -> ()  [unwired: 2 in, 2 out]
            n111 = call "Set Up Controls.vi"("error in"=w211) -> ("error out"=w205:errorcluster)  [unwired: 10 in]
            n112 = call "Set Up Accounts File.vi"("error in"=w205) -> ("error out"=w204:errorcluster)  [unwired: 10 in]
            n113 = call "Update ATM Messages.vi"("error in"=w204, "ATM Messages"="Welcome to Acme Bank. \nPlease insert your card \nand enter your account \nnumber in the User Input. \n \nPress Enter (E) when done. " ("Initial Message")) -> ("error out"=w210:errorcluster)  [unwired: 9 in]
            "Status" <- w213
          }
          frame "--- Private Requests ---" {
          }
          frame "Set Up Controls" {
            w235 = FALSE  # Disabled&GrayOut
            n114 = control-ref of="Card Simulator"() -> (w239:refnum<vi>)
            n115 = control-ref of="User Input"() -> (w246:refnum<vi>)
            n116 = control-ref of="Right Buttons"() -> (w245:refnum<vi>)
            n117 = control-ref of="Left Buttons"() -> (w244:refnum<vi>)
            n118 = control-ref of="Enter"() -> (w243:refnum<vi>)
            n119 = control-ref of="Left Menu"() -> (w242:refnum<vi>)
            n120 = control-ref of="Right Menu"() -> (w241:refnum<vi>)
            n121 = Build Array(w246, w245, w244, w243, w242, w241) -> (w240:refnum<vi>[])
            n122 = Bundle By Name(cluster=w249, "User Input ref"=w246, "Left Buttons ref"=w245, "Right Buttons ref"=w244, "Enter ref"=w243, "Right Menu ref"=w242, "Left Menu ref"=w241, "Card Simulator"=w239) -> (w248:T4)
            n123 = call "Enable or disable control or indicators.vi"("Enable (T)/Disable&GrayOut (F)"=w235, "error in (no error)"=w247, "aray of references in"=w240) -> ("error out"=w237:errorcluster, "Array of references dup"=w236:refnum<vi>[])  [unwired: 7 in]
            n124 = call "Get Controls Indicators Status by name.vi"("Enable (T)/Disable&GrayOut (F)"=w235, "error in (no error)"=w237, "aray of references"=w236) -> ("error out"=w233:errorcluster, "Status description"=w234:string)  [unwired: 7 in]
            n125 = call "Status Updated.vi"("error in"=w233, "Status"=w234) -> ("error out"=w238:errorcluster)  [unwired: 9 in]
          }
          frame "Set Up Accounts File" {
            n126 = Unbundle By Name(w257) -> ("Accounts.txt file name"=w254:string)
            n127 = call <vilib>:"Application Directory.vi"() -> ("Application Directory"=w255:path)
            n128 = Build Path(base path=w255, name or relative path=w254) -> (appended path=w251:path)
            n129 = call "Read Accounts Data.vi"("error in (no error)"=w253, "Accounts.txt file path"=w251) -> ("error out"=w252:errorcluster, "Accounts info"=w250:T6)  [unwired: 8 in]
            n130 = Bundle By Name(cluster=w257, "Accounts.txt file path"=w251, "Accounts info"=w250) -> (w256:T4)
          }
          frame "Update ATM Messages" {
            n131 = Variant To Data(error in=w264, type=T9 {"ATM Messages"=""} ("Update ATM Messages Argument"), Variant=w261) -> (data=w259:T9, error out=w262:errorcluster)
            n132 = Unbundle By Name(w259) -> ("ATM Messages"=→"ATM Messages":string)
          }
          frame "Verification OK" {
            w270 = FALSE  # Disable&GrayOut
            w283 = TRUE  # Enable
            # "The introduced value as a account number is correct"
            n133 = Unbundle By Name(w289) -> ("Account Info.Name"=w287:string, "Account Info.Surname"=w286:string, "Left Buttons ref"=w282:refnum<vi>, "Right Buttons ref"=w281:refnum<vi>, "Left Menu ref"=w274:refnum<vi>, "Right Menu ref"=w275:refnum<vi>, "Enter ref"=w269:refnum<vi>, "User Input ref"=w265:refnum<vi>)
            n134 = Build Array(w282, w281, w274, w275) -> (w284:refnum<vi>[])
            n135 = call "Prepare Left and Right Menus Strings.vi"("error in (no error)"=w277, "Right Menu ref"=w274, "Left Menu ref"=w275) -> ("error out"=w276:errorcluster)  [unwired: 8 in]
            n136 = Build Array(w269, w265) -> (w268:refnum<vi>[])
            n137 = call "Enable or disable control or indicators.vi"("Enable (T)/Disable&GrayOut (F)"=w283, "error in (no error)"=w276, "aray of references in"=w284) -> ("error out"=w267:errorcluster)  [unwired: 7 in, 1 out]
            n138 = invoke class="Str" method="Reinit To Default"(reference=w265, error in=w267) -> (error out=w266:errorcluster)  [unwired: 1 in, 2 out]
            n139 = Format Into String(format string="Welcome to Acme Bank \n%s %s\n \nPlease select transaction \nby using the buttons. ", w287, w286) -> (resulting string=w285:string)  [unwired: 2 in, 1 out]
            n140 = call "Enable or disable control or indicators.vi"("Enable (T)/Disable&GrayOut (F)"=w270, "error in (no error)"=w266, "aray of references in"=w268) -> ("error out"=w271:errorcluster)  [unwired: 7 in, 1 out]
            n141 = Bundle By Name(cluster=w289, "Verification OK?"=TRUE) -> (w273:T4)
            n142 = call "Update ATM Messages.vi"("error in"=w271, "ATM Messages"=w285) -> ("error out"=w280:errorcluster)  [unwired: 9 in]
            n143 = call "Start Timeout.vi"("error in"=w280, "Timeout Time (ms)"=10000) -> ("error out"=w279:errorcluster)  [unwired: 9 in]
          }
          frame "Verification NOK" {
            w293 = TRUE  # Key Focus
            # "Focuses the cursor to the User Input control"
            # "The introduced value as a account number is incorrect"
            n144 = Unbundle By Name(w294) -> ("User Input ref"=w290:refnum<vi>)
            n145 = property class="Str"(reference=w290, error in=w292, "Key Focus"=w293) -> (error out=w291:errorcluster)  [unwired: 1 out]
            n146 = call "Update ATM Messages.vi"("error in"=w291, "ATM Messages"="Account Information Incorrect \nPlease Re-Enter Account Number. \nPress Enter (E) when done ") -> ("error out"=w295:errorcluster)  [unwired: 9 in]
          }
          frame "Session Timed Out" {
            # "If the session is inactive for 10 seconds, stops the application (The message has already been sent)."
            n147 = call "Stop Module.vi"("error in"=w298) -> ("error out"=w297:errorcluster)  [unwired: 10 in]
          }
          frame "--- User Interface Events ---" {
            # "The following states are for user interface events"
          }
          frame "Update User Input" {
            # "Receive the User Input and stores it in the Main Cluster"
            n148 = Variant To Data(error in=w308, type="", Variant=w305) -> (data=w303:string, error out=w306:errorcluster)
            n149 = Bundle By Name(cluster=w307, "User Input"=w303) -> (w304:T4)
          }
          frame "Enter Button Pressed" {
            w314 = 10000  # Timeout Time (ms)
            # "Receive the User Input and stores it in the Main Cluster"
            n150 = Unbundle By Name(w321) -> ("Index of Account"=w310:i32, "Account Info"=w316:T5, "Accounts info"=w320:T6, "User Input"=w319:string, "Verification OK?"=w315:bool, "Pressed Button"=w311:string)
            n151 = case shown="True" w315 {
              tunnel: w322 -> [w328 w341]
              tunnel: w320 -> [w327 _]
              tunnel: w319 -> [w326 w338]
              tunnel: [w325 w340] -> w313
              tunnel: [w324 w342] -> w317
              tunnel: w316 -> [_ w342]
              tunnel: w311 -> [_ w339]
              tunnel: w310 -> [_ w335]
              tunnel: [w323 w335] -> w309
              frame False {
                n152 = call "Get Account Info.vi"("error in (no error)"=w328, "Account Number"=w326, "Accounts info"=w327) -> ("error out"=w329:errorcluster, "Valid Account?"=w330:bool, "Account Info"=w324:T5, "Index of Account"=w323:i32)  [unwired: 5 in]
                n153 = case shown="False" w330 {
                  tunnel: w329 -> [w332 w334]
                  tunnel: [w331 w333] -> w325
                  frame False {
                    # "The Account does not exist"
                    n154 = call "Verification NOK.vi"("error in"=w332) -> ("error out"=w331:errorcluster)  [unwired: 10 in]
                  }
                  frame True {
                    # "The Account Exists"
                    n155 = call "Verification OK.vi"("error in"=w334) -> ("error out"=w333:errorcluster)  [unwired: 10 in]
                  }
                }
              }
              frame True {
                w336 = u32 0  # u32
                # "Already checked, deposit introduced"
                n156 = Decimal String To Number(string=w338, default (0L)=w336) -> (number=w337:u32)  [unwired: 1 in, 1 out]
                n157 = case shown="\"Right Button Middle Pressed\"" w339 {
                  tunnel: w341 -> [w345 w346 w347 w350]
                  tunnel: [w343 w346 w347 w349] -> w340
                  tunnel: w337 -> [w344 _ _ w348]
                  frame "Right Button Middle Pressed" {
                    # "Withdraw"
                    n158 = call "Check Withdrawal.vi"("error in"=w345, "Withdraw Money"=w344) -> ("error out"=w343:errorcluster)  [unwired: 9 in]
                  }
                  frame "Right Button Bottom Pressed" {
                    # "Fast Cash $50"
                  }
                  frame Default {
                  }
                  frame "Right Button Top Pressed" {
                    # "Deposit"
                    n159 = call "Deposit Introduced.vi"("error in"=w350, "Deposit Money"=w348) -> ("error out"=w349:errorcluster)  [unwired: 9 in]
                  }
                }
              }
            }
            n160 = Bundle By Name(cluster=w321, "Account Info"=w317, "Index of Account"=w309) -> (w318:T4)
            n161 = call "Start Timeout.vi"("error in"=w313, "Timeout Time (ms)"=w314) -> ("error out"=w312:errorcluster)  [unwired: 9 in]
          }
          frame "Card Simulator Button Pressed" {
            w361 = TRUE  # Key Focus
            w352 = TRUE  # Enabled
            # "Focuses the cursor to the User Input control"
            n162 = Unbundle By Name(w364) -> ("User Input ref"=w360:refnum<vi>, "Enter ref"=w363:refnum<vi>)
            n163 = Build Array(w360, w363) -> (w366:refnum<vi>[])
            n164 = Merge Errors(w365) -> (w362:errorcluster)
            n165 = call "Enable or disable control or indicators.vi"("Enable (T)/Disable&GrayOut (F)"=w352, "error in (no error)"=w362, "aray of references in"=w366) -> ("error out"=w356:errorcluster, "Array of references dup"=w353:refnum<vi>[])  [unwired: 7 in]
            n166 = call "Get Controls Indicators Status by name.vi"("Enable (T)/Disable&GrayOut (F)"=w352, "error in (no error)"=w356, "aray of references"=w353) -> ("error out"=w355:errorcluster, "Status description"=w357:string)  [unwired: 7 in]
            n167 = call "Status Updated.vi"("error in"=w355, "Status"=w357) -> ("error out"=w354:errorcluster)  [unwired: 9 in]
            n168 = property class="Str"(reference=w360, error in=w354, "Key Focus"=w361) -> (error out=w351:errorcluster)  [unwired: 1 out]
            n169 = call "Start Timeout.vi"("error in"=w351, "Timeout Time (ms)"=10000) -> ("error out"=w358:errorcluster)  [unwired: 9 in]
          }
          frame "Right Button Top Pressed" {
            w369 = 10000  # Timeout Time (ms)
            w377 = TRUE  # Enabled
            # "Deposit button pressed"
            n170 = Unbundle By Name(w376) -> ("Enter ref"=w375:refnum<vi>, "User Input ref"=w374:refnum<vi>)
            n171 = call "Update ATM Messages.vi"("error in"=w378, "ATM Messages"="Please enter amount to deposit and press \nEnter (E) when done ") -> ("error out"=w372:errorcluster)  [unwired: 9 in]
            n172 = Bundle By Name(cluster=w376, "Pressed Button"=w367) -> (w368:T4)
            n173 = Build Array(w375, w374) -> (w373:refnum<vi>[])
            n174 = call "Enable or disable control or indicators.vi"("Enable (T)/Disable&GrayOut (F)"=w377, "error in (no error)"=w372, "aray of references in"=w373) -> ("error out"=w371:errorcluster)  [unwired: 7 in, 1 out]
            n175 = call "Start Timeout.vi"("error in"=w371, "Timeout Time (ms)"=w369) -> ("error out"=w370:errorcluster)  [unwired: 9 in]
          }
          frame "Right Button Middle Pressed" {
            w388 = TRUE  # Enabled
            w392 = 10000  # Timeout Time (ms)
            # "Withdraw button pressed"
            n176 = Unbundle By Name(w384) -> ("Enter ref"=w386:refnum<vi>, "User Input ref"=w385:refnum<vi>)
            n177 = Build Array(w386, w385) -> (w383:refnum<vi>[])
            n178 = call "Enable or disable control or indicators.vi"("Enable (T)/Disable&GrayOut (F)"=w388, "error in (no error)"=w387, "aray of references in"=w383) -> ("error out"=w382:errorcluster)  [unwired: 7 in, 1 out]
            n179 = Bundle By Name(cluster=w384, "Pressed Button"=w389) -> (w390:T4)
            n180 = call "Update ATM Messages.vi"("error in"=w382, "ATM Messages"="Please enter amount to withdraw and press \nEnter (E) when done") -> ("error out"=w381:errorcluster)  [unwired: 9 in]
            n181 = call "Start Timeout.vi"("error in"=w381, "Timeout Time (ms)"=w392) -> ("error out"=w391:errorcluster)  [unwired: 9 in]
          }
          frame "Left Button Middle Pressed" {
            w402 = 10000  # Timeout Time (ms)
            # "Withdraw button pressed"
            n182 = Unbundle By Name(w396) -> ("Account Info.Remaining Money"=w394:i32)
            n183 = Format Into String(format string="Your Balance Is: \n$%d" ("ATM Messages"), w394) -> (resulting string=w393:string)  [unwired: 2 in, 1 out]
            n184 = Bundle By Name(cluster=w396, "Pressed Button"=w399) -> (w400:T4)
            n185 = call "Update ATM Messages.vi"("error in"=w398, "ATM Messages"=w393) -> ("error out"=w397:errorcluster)  [unwired: 9 in]
            n186 = call "Start Timeout.vi"("error in"=w397, "Timeout Time (ms)"=w402) -> ("error out"=w401:errorcluster)  [unwired: 9 in]
          }
          frame "Right Button Bottom Pressed" {
            w411 = TRUE  # Enabled
            w415 = 10000  # Timeout Time (ms)
            # "Fast Cash $50 button pressed"
            n187 = Unbundle By Name(w407) -> ("Enter ref"=w409:refnum<vi>, "User Input ref"=w408:refnum<vi>)
            n188 = Build Array(w409, w408) -> (w406:refnum<vi>[])
            n189 = Bundle By Name(cluster=w407, "Pressed Button"=w412) -> (w413:T4)
            n190 = call "Enable or disable control or indicators.vi"("Enable (T)/Disable&GrayOut (F)"=w411, "error in (no error)"=w410, "aray of references in"=w406) -> ("error out"=w404:errorcluster)  [unwired: 7 in, 1 out]
            n191 = call "Deposit Introduced.vi"("error in"=w404, "Deposit Money"=u32 50) -> ("error out"=w403:errorcluster)  [unwired: 9 in]
            n192 = call "Start Timeout.vi"("error in"=w403, "Timeout Time (ms)"=w415) -> ("error out"=w414:errorcluster)  [unwired: 9 in]
          }
          frame "Left Button Bottom Pressed" {
            # "Return Card & Terminate button pressed"
            n193 = Unbundle By Name(w420) -> ("Card Simulator"=w416:refnum<vi>)
            n194 = Bundle By Name(cluster=w420, "Pressed Button"=w421) -> (w422:T4)
            n195 = invoke class="Bool" method="Reinit To Default"(reference=w416, error in=w418) -> (error out=w417:errorcluster)  [unwired: 1 in, 2 out]
            n196 = call "Stop Module.vi"("error in"=w417) -> ("error out"=w419:errorcluster)  [unwired: 10 in]
          }
          frame "Deposit Introduced" {
            w436 = FALSE  # Disable&GrayOut
            n197 = Variant To Data(error in=w444, type=T8 {"Deposit Money"=0} ("Deposit Introduced Argument"), Variant=w443) -> (data=w441:T8, error out=w425:errorcluster)
            n198 = Unbundle By Name(w440) -> ("Account Info.Remaining Money"=w439:i32, "Enter ref"=w435:refnum<vi>, "User Input ref"=w423:refnum<vi>)
            n199 = Unbundle By Name(w441) -> ("Deposit Money"=w430:u32)
            n200 = Add(x=w439, y=w430) -> (x+y=w437:u32)
            n201 = invoke class="Str" method="Reinit To Default"(reference=w423, error in=w425) -> (error out=w424:errorcluster)  [unwired: 1 in, 2 out]
            n202 = Format Into String(format string="$%d Deposited", error in=w424, w430) -> (resulting string=w433:string, error out=w429:errorcluster)  [unwired: 1 in]
            n203 = Bundle By Name(cluster=w440, "Account Info.Remaining Money"=w437) -> (w438:T4)
            n204 = Build Array(w435, w423) -> (w434:refnum<vi>[])
            n205 = call "Update ATM Messages.vi"("error in"=w429, "ATM Messages"=w433) -> ("error out"=w431:errorcluster)  [unwired: 9 in]
            n206 = call "Enable or disable control or indicators.vi"("Enable (T)/Disable&GrayOut (F)"=w436, "error in (no error)"=w431, "aray of references in"=w434) -> ("error out"=w427:errorcluster)  [unwired: 7 in, 1 out]
            n207 = call "Save Account.vi"("error in"=w427) -> ("error out"=w426:errorcluster)  [unwired: 10 in]
            n208 = call "Stop Timeout.vi"("error in"=w426) -> ("error out"=w428:errorcluster)  [unwired: 10 in]
          }
          frame "Save Account" {
            n209 = Unbundle By Name(w452) -> ("Index of Account"=w445:i32, "Accounts.txt file path"=w451:path, "Accounts info"=w450:T6, "Account Info"=w449:T5)
            n210 = call "Write Accounts info.vi"("Index of Account"=w445, "error in (no error)"=w453, "Account Info"=w449, "Accounts info in"=w450, "Accounts.txt file path"=w451) -> ("error out"=w448:errorcluster, "Accounts info out"=w446:T6)  [unwired: 5 in]
            n211 = Bundle By Name(cluster=w452, "Accounts info"=w446) -> (w447:T4)
          }
          frame "Check Withdrawal" {
            n212 = Variant To Data(error in=w468, type=T7 {"Withdraw Money"=0} ("Check Withdrawal Argument"), Variant=w467) -> (data=w465:T7, error out=w463:errorcluster)
            n213 = Unbundle By Name(w459) -> ("Enter ref"=w455:refnum<vi>, "User Input ref"=w454:refnum<vi>, "Account Info.Remaining Money"=w464:i32)
            n214 = Unbundle By Name(w465) -> ("Withdraw Money"=w460:i32)
            n215 = Subtract(x=w464, y=w460) -> (x-y=w458:i32)
            n216 = To Long Integer(number=w458) -> (32bit integer=w456:i32)
            n217 = Less Than 0?(x=w456) -> (x < 0?=w461:bool)
            n218 = case shown="False" w461 {
              tunnel: w463 -> [w472 w487]
              tunnel: [w475 w486] -> w462
              tunnel: w460 -> [w482 _]
              tunnel: w459 -> [w481 w484]
              tunnel: w456 -> [w480 _]
              tunnel: [w479 w484] -> w457
              tunnel: w455 -> [w473 _]
              tunnel: w454 -> [w470 _]
              frame False {
                w477 = FALSE  # Disable&GrayOut
                n219 = invoke class="Str" method="Reinit To Default"(reference=w470, error in=w472) -> (error out=w471:errorcluster)  [unwired: 1 in, 2 out]
                n220 = Format Into String(format string="$%d Withdrawn ", w482) -> (resulting string=w469:string)  [unwired: 2 in, 1 out]
                n221 = call "Update ATM Messages.vi"("error in"=w471, "ATM Messages"=w469) -> ("error out"=w478:errorcluster)  [unwired: 9 in]
                n222 = call "Save Account.vi"("error in"=w478) -> ("error out"=w476:errorcluster)  [unwired: 10 in]
                n223 = Bundle By Name(cluster=w481, "Account Info.Remaining Money"=w480) -> (w479:T4)
                n224 = Build Array(w473, w470) -> (w474:refnum<vi>[])
                n225 = call "Enable or disable control or indicators.vi"("Enable (T)/Disable&GrayOut (F)"=w477, "error in (no error)"=w476, "aray of references in"=w474) -> ("error out"=w475:errorcluster)  [unwired: 7 in, 1 out]
              }
              frame True {
                n226 = call "Update ATM Messages.vi"("error in"=w487, "ATM Messages"="Insufficient funds in account \nPlease check your balance \nand try again ") -> ("error out"=w486:errorcluster)  [unwired: 9 in]
              }
            }
          }
          frame "---Testing Requests---" {
            # "The following states are for testing purposes only"
            n227 = Merge Errors(w490) -> (w489:errorcluster)
          }
          frame "Testing - Update ATM Messages" {
            # "This state is for testing the Update ATM Messages request"
            n228 = call "Update ATM Messages.vi"("error in"=w495, "ATM Messages"="Welcome to Acme Bank. \nThis message is for testing purposes only. " ("Initial Message")) -> ("error out"=w493:errorcluster)  [unwired: 9 in]
            n229 = call "Status Updated.vi"("error in"=w493, "Status"="Testing MSG shown in the ATM Messages box.") -> ("error out"=w492:errorcluster)  [unwired: 9 in]
          }
          frame "Testing - Generate File Not Found Error" {
            # "This request is for testing purposes only, it generates an error 7 (File not found) in order to check that the error management is correct."
            n230 = xnode "Error Ring"() -> ("error out"=w497:errorcluster)
            n231 = Merge Errors(w499, w497) -> (w498:errorcluster)
          }
          frame "Testing - Enable All Elements in FP" {
            w518 = TRUE  # Enable
            # "This request is for testing purposes only, it enables all the elements in the Front Panel using its requests stored in the Module Data Cluster"
            n232 = Unbundle By Name(w513) -> ("User Input ref"=w512:refnum<vi>, "Left Buttons ref"=w511:refnum<vi>, "Right Buttons ref"=w510:refnum<vi>, "Enter ref"=w509:refnum<vi>, "Right Menu ref"=w508:refnum<vi>, "Left Menu ref"=w507:refnum<vi>, "Card Simulator"=w506:refnum<vi>)
            n233 = Build Array(w512, w511, w510, w509, w508, w507, w506) -> (w505:refnum<vi>[])
            n234 = call "Enable or disable control or indicators.vi"("Enable (T)/Disable&GrayOut (F)"=w518, "error in (no error)"=w515, "aray of references in"=w505) -> ("error out"=w520:errorcluster, "Array of references dup"=w519:refnum<vi>[])  [unwired: 7 in]
            n235 = call "Get Controls Indicators Status by name.vi"("Enable (T)/Disable&GrayOut (F)"=w518, "error in (no error)"=w520, "aray of references"=w519) -> ("error out"=w516:errorcluster, "Status description"=w517:string)  [unwired: 7 in]
            n236 = call "Status Updated.vi"("error in"=w516, "Status"=w517) -> ("error out"=w514:errorcluster)  [unwired: 9 in]
          }
          frame "Testing - Disable All Elements in FP" {
            w534 = FALSE  # Disabled&GrayOut
            # "This request is for testing purposes only, it enables all the elements in the Front Panel using its requests stored in the Module Data Cluster"
            n237 = Unbundle By Name(w529) -> ("User Input ref"=w528:refnum<vi>, "Left Buttons ref"=w527:refnum<vi>, "Right Buttons ref"=w526:refnum<vi>, "Enter ref"=w525:refnum<vi>, "Right Menu ref"=w524:refnum<vi>, "Left Menu ref"=w523:refnum<vi>, "Card Simulator"=w522:refnum<vi>)
            n238 = Build Array(w528, w527, w526, w525, w524, w523, w522) -> (w521:refnum<vi>[])
            n239 = call "Enable or disable control or indicators.vi"("Enable (T)/Disable&GrayOut (F)"=w534, "error in (no error)"=w531, "aray of references in"=w521) -> ("error out"=w536:errorcluster, "Array of references dup"=w535:refnum<vi>[])  [unwired: 7 in]
            n240 = call "Get Controls Indicators Status by name.vi"("Enable (T)/Disable&GrayOut (F)"=w534, "error in (no error)"=w536, "aray of references"=w535) -> ("error out"=w532:errorcluster, "Status description"=w533:string)  [unwired: 7 in]
            n241 = call "Status Updated.vi"("error in"=w532, "Status"=w533) -> ("error out"=w530:errorcluster)  [unwired: 9 in]
          }
          frame "---Exit and Error Handling---" {
            # "Separator - The following cases handle errors and exit messages."
          }
          frame "Error" {
            # "This module is going to be launched always in non external"
            # "Error - Check the error message data and respond accordingly. This message is sent by the \"Error Handler\" VIs at the end of each loop in this application."
            n242 = property on="Property Node" class="Module Admin" props=["Accessors:External Launch"](reference=w541) -> ()  [unwired: 1 in, 3 out]
            n243 = Variant To Data(error in=w549, type=errorcluster {"status"=FALSE, "code"=0, "source"=""} ("error constant"), Variant=w543) -> (data=w540:errorcluster, error out=w547:errorcluster)
            n244 = local write "error out"(w540) -> ()
            n245 = call "Error Reported.vi"("Error"=w540) -> ()  [unwired: 10 in, 1 out]
            n246 = case shown="False" FALSE {
              tunnel: [w554 _] -> w546
              tunnel: w542 -> [w552 _]
              tunnel: w540 -> [w553 _]
              frame False {
                n247 = disable-structure shown="Default" {
                  disable-tunnel: w553 -> [w555 _]
                  frame condition #0 (active) {
                    # "If the module is running standalone, then pop up an error dialog and call the \"Exit\" message."
                    n248 = call <vilib>:"Simple Error Handler.vi"("error in (no error)"=w555) -> ()  [unwired: 4 in, 5 out]
                  }
                  frame condition #1 {
                    # "To prevent the Simple Error Handler VI from being loaded (e.g. when deploying to a Real-Time target), add the Conditional Disable Symbol \"DQMH_Disable_SEH\" to your project and set it to TRUE."
                  }
                }
                n249 = call-poly <vilib>:"Delacor_lib_QMH_Enqueue Message (poly).vi"("Priority Message? (F)"=TRUE, "Message"="Exit", "Message Queue in"=w552) -> ("error out"=w554:errorcluster)  [unwired: 7 in, 1 out]
              }
              frame True {
                # "If the module was launched externally, calling the Error Reported broadcast VI is the only action performed by the \"Error\" message. The module's caller can then process the error appropriately."
              }
            }
            n250 = Merge Errors(w547, w546) -> (w545:errorcluster)
          }
          frame "Exit" {
            w561 = 91  # 91: not all Exit messages will have an argument
            w563 = TRUE  # Stop the VI
            # "Release the message queue reference"
            # "#DQMH_CodeNeeded - Add any required cleanup code here."
            # "Exit - Exit the application."
            n251 = Variant To Data(error in=w571, type=T11 {"Origin"="", "Exit via Stop Module Req?"=FALSE, "Wait for Module to stop?"=FALSE} ("Stop Argument"), Variant=w562) -> (data=w559:T11, error out=w568:errorcluster)
            n252 = call <vilib>:"Clear Errors.vi"("error in (no error)"=w568, "specific error code to clear (0: all)"=w561) -> ("error out"=w570:errorcluster)  [unwired: 4 in, 1 out]
            n253 = control-ref of="This VI"() -> (w558:refnum<vi>)
            n254 = call-dynamic "Delacor_lib_QMH_Release Message Queue.vi"("error in"=w570, "Message Queue"=w565) -> ("error out"=w569:errorcluster)  [unwired: 9 in]
            n255 = call "Handle Exit.vi"("Stop Argument"=w559, "Admin in"=w557, "VI reference"=w558) -> ("error out"=w567:errorcluster)  [unwired: 7 in, 1 out]
            n256 = Merge Errors(w569, w567) -> (w566:errorcluster)
            n257 = call "Error Reported.vi"("Error"=w566) -> ()  [unwired: 10 in, 1 out]
            n258 = local write "ATM Messages"("Your session has been terminated \ndue to inactivity or menu selection. \nPlease take your card \n \nGoodbye!") -> ()
          }
          frame Default {
            # "'Default' case only runs if there is a message that isn't defined in any of the other cases.  Output a programming error."
            n259 = call "Module Name--constant.vi"() -> ("Module Name"=w576:string)  [unwired: 11 in]
            n260 = Format Into String(format string="The invalid message string \"%s\" was received in the Message Handling Loop for module \"%s\".", w577, w576) -> (resulting string=w572:string)  [unwired: 2 in, 1 out]
            n261 = call <vilib>:"Error Cluster From Error Code.vi"("show call chain? (False)"=TRUE, "error message (\"\")"=w572, "error code (0)"=1) -> ("error out"=w579:errorcluster)  [unwired: 6 in]
            n262 = Merge Errors(w580, w579) -> (w581:errorcluster)
          }
        }
        n263 = call-dynamic "Delacor_lib_QMH_Error Handler - Message Handling Loop.vi"("error in"=w194, "Message Queue in"=w193) -> ("dup error in"=w195:errorcluster)  [unwired: 8 in, 1 out]
      }
    }
    frame Error {
      # "Synchronize Caller Events.vi will inform Start Module.vi that the module has launched and will let the code calling Start Module.vi register for broadcasts and would permit the caller receive the broadcast that an error occurred at launch time."
      n264 = call-dynamic "Delacor_lib_QMH_Release Message Queue.vi"("error in"=w589, "Message Queue"=w582) -> ("error out"=w588:errorcluster)  [unwired: 9 in]
      n265 = call "Synchronize Caller Events.vi"("Singleton Module Admin in"=w583) -> ("error out"=w590:errorcluster)  [unwired: 9 in, 1 out]
      n266 = call "Module Name--constant.vi"() -> ("Module Name"=w586:string)  [unwired: 11 in]
      n267 = Format Into String(format string="An error occurred during initialization. %s is no longer running.", w586) -> (resulting string=w584:string)  [unwired: 2 in, 1 out]
      n268 = Merge Errors(w588, w590) -> (w591:errorcluster)
      n269 = call "Error Reported.vi"("Additional Information"=w584, "Error"=w591) -> ()  [unwired: 9 in, 1 out]
    }
  }
  n270 = Merge Errors(w14, w17) -> (w13:errorcluster)
  n271 = call "Close Module.vi"("error in"=w13, "Module Admin in"=w8) -> ("error out"=w15:errorcluster, "External Launch"=w1:bool, "Module Admin out"=w2:refnum<class "Delacor_lib_QMH_Module Admin.lvclass">)  [unwired: 7 in]
  n272 = Unregister For Events(event registration refnum=w7, error in=w15) -> (error out=w12:errorcluster)
  "error out" <- w12
  n273 = case "External Launch?" shown="True" w1 {
    tunnel: w12 -> [_ w592]
    frame False {
    }
    frame True {
      n274 = case shown="No Error" w592 {
        frame No Error {
          n275 = invoke on="Invoke Node" class="VI" method="FP.Close"() -> ()  [unwired: 3 in, 3 out]
        }
        frame Error {
          n276 = disable-structure shown="Default" {
            frame condition #0 (active) {
              n277 = invoke class="VI" method="FP.Open"("Activate"=TRUE ("Activate?")) -> ()  [unwired: 4 in, 5 out]
            }
            frame condition #1 {
              # "Don't show panel on error if running inside a built EXE."
            }
          }
        }
      }
    }
  }
  n278 = local write "Module Admin"(w2) -> ()
